vi "Add_ID_and_Length.vi"(9 "PayldLen":u32, 10 "Signal Settings In":T1[](array[typedef]) {"Protection Configuration"."CRC Channels"."Data Type" items=["Signed", "Unsigned", "IEEE Float"]}, 11 "ID":u32) -> (2 "Signal Settings Out":T1[](array[typedef]) {"Protection Configuration"."CRC Channels"."Data Type" items=["Signed", "Unsigned", "IEEE Float"]})   [LabVIEW 2015, in "Protection and Counter Support System Explorer.lvlib"]
doc: "For each signal in the frame, this VI adds the appropriate frame ID and payload length"
uses:
  Protection and Counter Support System Explorer.lvlib
  Shared/Types/Exported Signal Settings.ctl
  Shared/Types/Exported Counter Settings.ctl
  Shared/Types/Exported Protection Settings.ctl
  Shared/Types/Protection Type.ctl
  Shared/Types/XNET Signal Configuration.ctl
  Shared/Protection and Counter Support Shared.lvlib
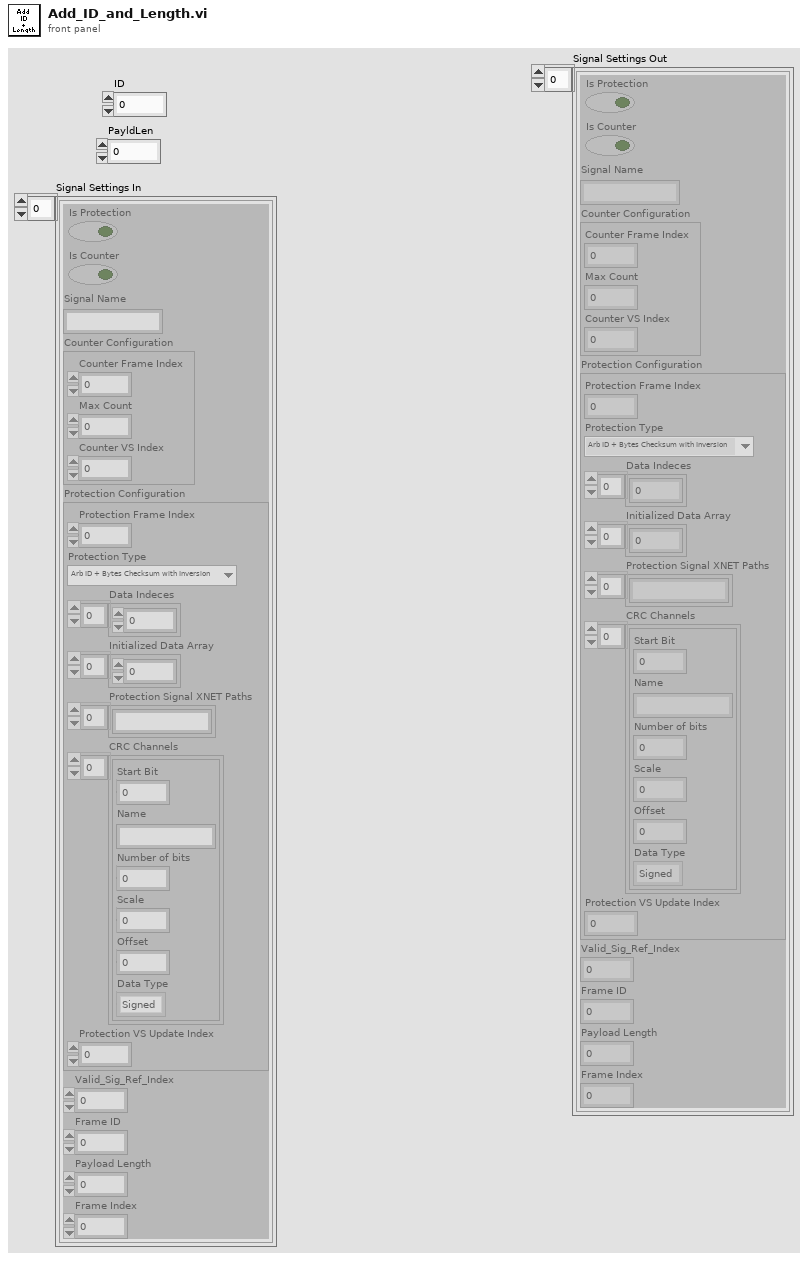
[diagram p1: front panel]
types:
  T1 = typedef "Protection and Counter Support Shared.lvlib/Exported Signal Settings.ctl" = cluster{"Is Protection":bool, "Is Counter":bool, "Signal Name":string, "Counter Configuration":T2, "Protection Configuration":T3, "Valid_Sig_Ref_Index":i32, "Frame ID":u32, "Payload Length":u32, "Frame Index":i32}
  T2 = typedef "Protection and Counter Support Shared.lvlib/Exported Counter Settings.ctl" = cluster{"Counter Frame Index":i32, "Max Count":dbl, "Counter VS Index":i32}
  T3 = typedef "Protection and Counter Support Shared.lvlib/Exported Protection Settings.ctl" = cluster{"Protection Frame Index":i32, "Protection Type":T4, "Data Indeces":i32[], "Initialized Data Array":dbl[], "Protection Signal XNET Paths":string[], "CRC Channels":T5[], "Protection VS Update Index":i32}
  T4 = typedef "Protection and Counter Support Shared.lvlib/Protection Type.ctl" = enum16{"Arb ID + Bytes Checksum with Inversion", "Arb ID + Bytes CRC with Inversion (Little Endian Only)", "Reversed Raw Signal Checksum with Inversion"}
  T5 = typedef "Protection and Counter Support Shared.lvlib/XNET Signal Configuration.ctl" = cluster{"Start Bit":i32, "Name":string, "Number of bits":i32, "Scale":dbl, "Offset":dbl, "Data Type":u32}
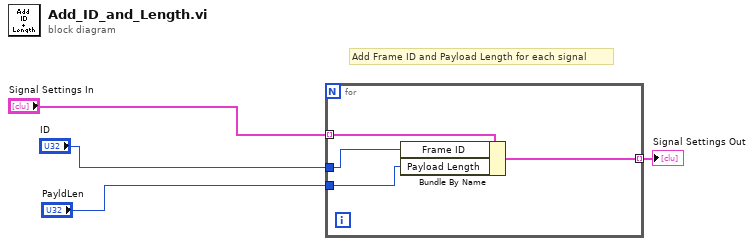
[diagram p0: block diagram]
diagram:
  # "Add Frame ID and Payload Length for each signal"
  n1 = for {
    tunnel: "Signal Settings In" -> [w8] mode=indexing
    tunnel: "ID" -> [w7]
    tunnel: "PayldLen" -> [w6]
    tunnel: [w5] -> w1 mode=indexing
    n2 = Bundle By Name(cluster=w8, "Frame ID"=w7, "Payload Length"=w6) -> (w5:T1)
  }
  "Signal Settings Out" <- w1
